vi "FiberSpectrograph_acceptCommand_setValue.vi"(8 "error in (no error)":errorcluster, 11 "command_setValue_Ctl":T1) -> (0 "error out":errorcluster, 2 "function return":i32, 3 "command_setValue_Ctl out":T1)   [LabVIEW 2016, in "SALLV_FiberSpectrograph.lvlib"]
doc: "int FiberSpectrograph_shm_acceptCommand_setValueLV(FiberSpectrograph_command_setValueLV *command_setValue_Ctl );"
uses:
  SALLV_FiberSpectrograph.lvlib
  DataTypes/command_setValue.ctl
  SALLV_FiberSpectrograph.so
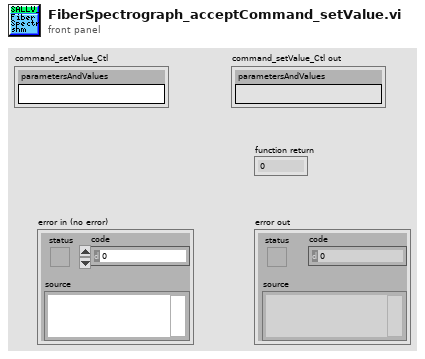
[diagram p1: front panel]
types:
  T1 = typedef "SALLV_FiberSpectrograph.lvlib/command_setValue.ctl" = cluster{"parametersAndValues":string}
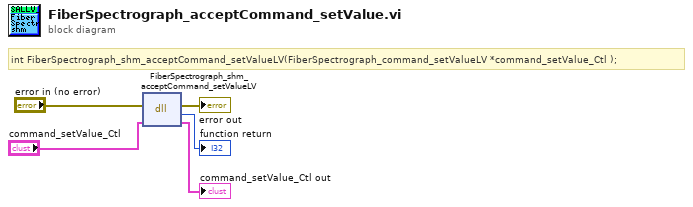
[diagram p0: block diagram]
diagram:
  # "int FiberSpectrograph_shm_acceptCommand_setValueLV(FiberSpectrograph_command_setValueLV *command_setValue_Ctl );"
  n1 = dll-call lib="home/harini/tcs/sallv_FiberSpectrometer/SALLV_FiberSpectrograph.*" fn="FiberSpectrograph_shm_acceptCommand_setValueLV"(error in="error in (no error)", "command_setValue_Ctl"="command_setValue_Ctl") -> (error out=→"error out":errorcluster, →"function return":i32, "command_setValue_Ctl"=→"command_setValue_Ctl out":T1)  [unwired: 2 in, 1 out]
